vi "Actor Core.vi"(8 "error in":errorcluster, 11 "Explain Error Improved Dialog in":refnum<class "Explain Error Improved Dialog.lvclass">) -> (0 "error out":errorcluster, 3 "Actor out":refnum<class "Actor.lvclass">)   [LabVIEW 2020, in "Explain Error Improved Dialog.lvlib" / "Explain Error Improved Dialog.lvclass"]
doc: "(<B>Filename</B>: Actor Framework.lvlib:Actor.lvclass:Actor Core.vi)\n\nReceives messages to the actor, reacts to them, and initiates any error handling that may shut the actor down.\n\nDescendant classes may override this VI to append parallel tasks for the actor to complete while it handles messages. Overrides use the Call Parent Class Method node."
uses:
  <resource>/plugins/PopupMenus/edit time panel and diagram/Explain Error (Improved)/Explain Error Improved Dialog/Explain Error Improved Dialog/Explain Error Improved Dialog.lvclass
  C:/Program Files/National Instruments/LabVIEW 2020/vi.lib/ActorFramework/Actor/Actor.lvclass
  <vilib>/ActorFramework/Actor/Actor.lvclass
  <resource>/plugins/PopupMenus/edit time panel and diagram/Explain Error (Improved)/Explain Error Improved Dialog/Explain Error Improved Dialog/Explain Error Improved Dialog.lvclass/Explain Error Improved Dialog.ctl
  <vilib>/ActorFramework/Actor/Actor.lvclass/Actor.ctl
  <vilib>/ActorFramework/Message Enqueuer/Message Enqueuer.lvclass/Message Enqueuer.ctl
  <vilib>/ActorFramework/Message Enqueuer/Init from Existing Queue.vi
  <vilib>/ActorFramework/Message Enqueuer/Enqueue.vi
  <vilib>/ActorFramework/Stop Msg/Stop Msg.lvclass
  C:/Program Files/National Instruments/LabVIEW 2020/vi.lib/ActorFramework/Message/Message.lvclass
  <vilib>/ActorFramework/Message Priority Queue/Priority Enqueue.vi
  <vilib>/ActorFramework/Message Enqueuer/Message Enqueuer.lvclass
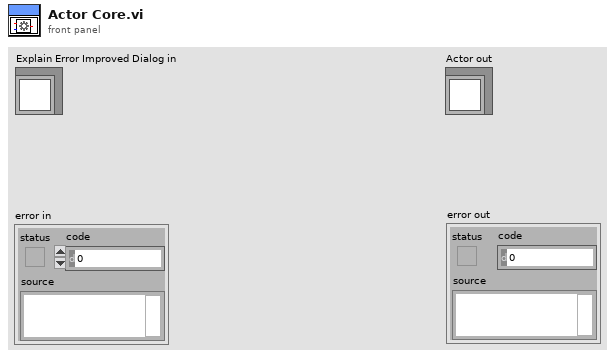
[diagram p1: front panel]
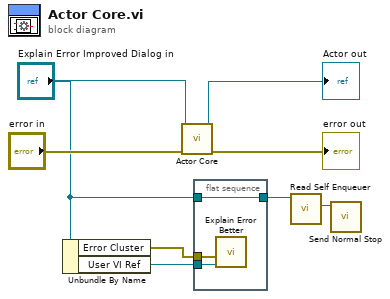
[diagram p0: block diagram]
diagram:
  n1 = Unbundle By Name("Explain Error Improved Dialog in") -> ("Error Cluster"=w4:errorcluster, "User VI Ref"=w5:refnum<vi>)
  n2 = call-parent "Actor Core.vi"("error in"="error in", "Actor in"="Explain Error Improved Dialog in") -> ("error out"=→"error out":errorcluster, "Actor out"=→"Actor out":refnum<class "Actor.lvclass">)  [unwired: 8 in]
  n3 = flat-sequence {
    tunnel: w5 -> [w11]
    tunnel: w4 -> [w10]
    tunnel: [w9] -> w1
    tunnel: "Explain Error Improved Dialog in" -> [w9]
    frame #0 {
      n4 = call <resource>:"Explain Error Better.vi"("User VI Ref"=w11, "Error Cluster"=w10) -> ()  [unwired: 10 in]
    }
  }
  n5 = call <vilib>:"Read Self Enqueuer.vi"("Actor"=w1) -> ("Self Enqueuer"=w2:refnum<class "Message Enqueuer.lvclass">)  [unwired: 10 in]
  n6 = call <vilib>:"Send Normal Stop.vi"("Message Enqueuer"=w2) -> ()  [unwired: 10 in, 1 out]
